vi "delete duplicates.vi"(9 "After Var Name":string[](array[string]), 10 "subscripts":string[](array[string]), 11 "Name":string[](array[string])) -> (0 "After Var Name Out":string[](array[string]), 1 "Full Names":string[][](array[string]), 2 "Subscripts Out":string[][](array[string]), 3 "Name Out":string[](array[string]), 4 "Name.Sub":string[](array[string]))   [LabVIEW 2015, in "AguaClara Library.lvlib"]
uses:
  ADT 2/AguaClara Library.lvlib
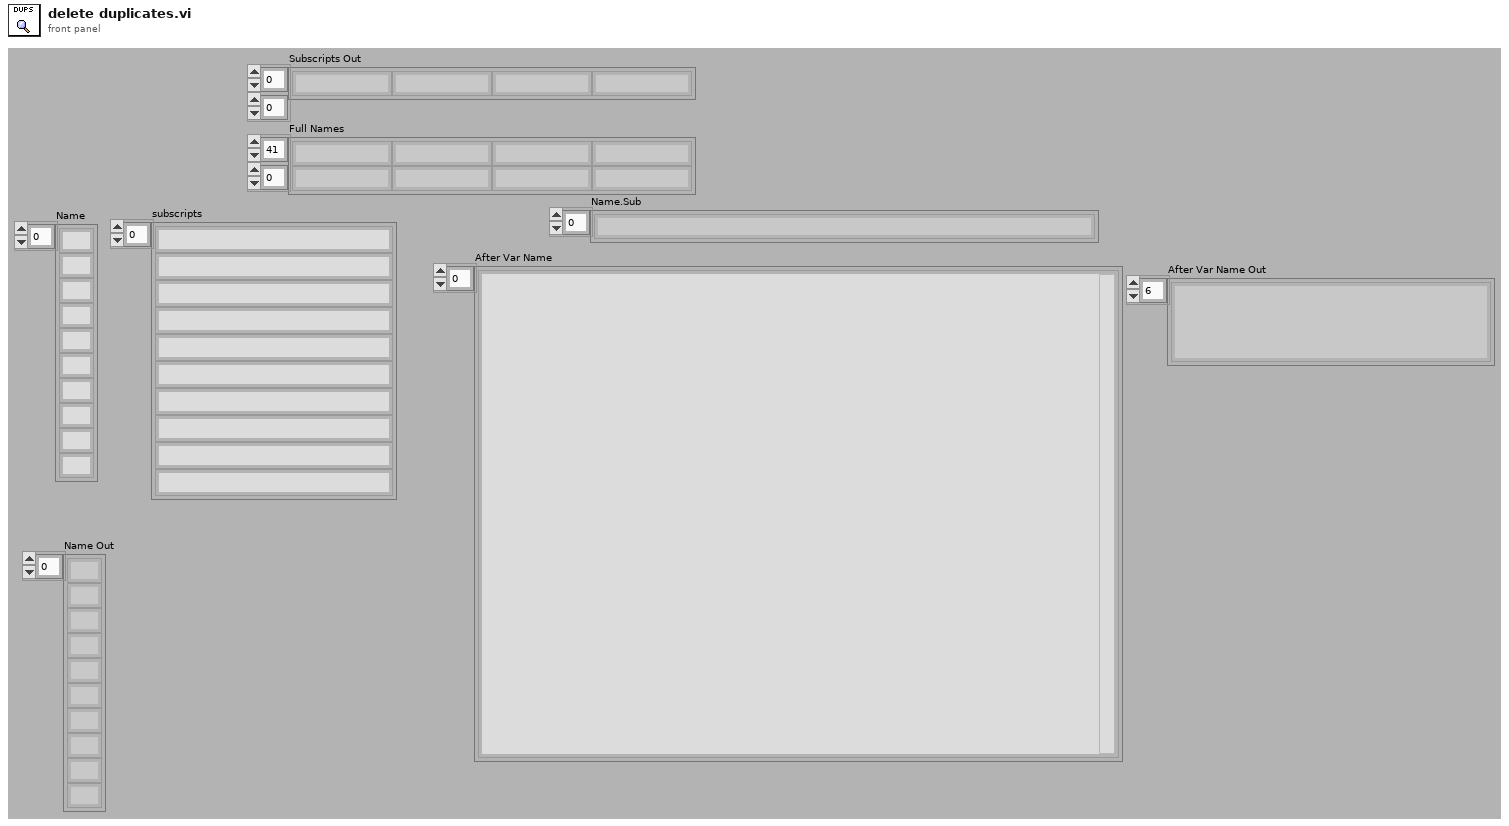
[diagram p1: front panel]
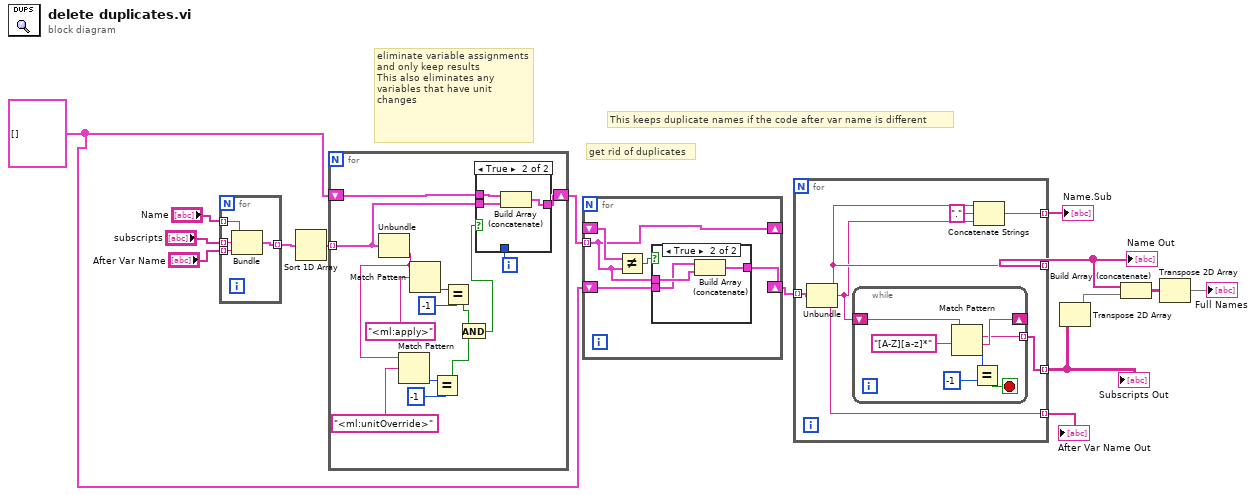
[diagram p0: block diagram]
diagram:
  w1 = cluster{string, string, "XML":string}[] []
  # "eliminate variable assignments and only keep results\nThis also eliminates any variables that have unit changes"
  # "This keeps duplicate names if the code after var name is different"
  # "get rid of duplicates"
  n1 = for {
    tunnel: "Name" -> [w19] mode=indexing
    tunnel: "subscripts" -> [w18] mode=indexing
    tunnel: [w17] -> w13 mode=indexing
    tunnel: "After Var Name" -> [w16] mode=indexing
    n2 = Bundle(w19, w18, "XML"=w16) -> (w17:cluster{string, string, "XML":string})  [unwired: 1 in]
  }
  n3 = Sort 1D Array(array=w13) -> (sorted array=w3:cluster{string, string, "XML":string}[])
  n4 = for {
    tunnel: w3 -> [w30] mode=indexing
    shift-right: [w29] -> w2
    shift-left: w1 -> [w28]
    i -> [w31]
    n5 = Unbundle(w30) -> ("XML"=w23:string)  [unwired: 2 out]
    n6 = Match Pattern(string=w23, regular expression="<ml:unitOverride>") -> (offset past match=w26:i32)  [unwired: 1 in, 3 out]
    n7 = Match Pattern(string=w23, regular expression="<ml:apply>") -> (offset past match=w33:i32)  [unwired: 1 in, 3 out]
    n8 = Equal?(x=w26, y=-1) -> (x = y?=w22:bool)
    n9 = Equal?(x=w33, y=-1) -> (x = y?=w21:bool)
    n10 = And(x=w21, y=w22) -> (x .and. y?=w20:bool)
    n11 = case shown="True" w20 {
      tunnel: w31 -> [_ _]
      tunnel: w30 -> [_ w37]
      tunnel: [w34 w36] -> w29
      tunnel: w28 -> [w34 w35]
      frame False {
      }
      frame True {
        n12 = Build Array (concatenate)(w35, w37) -> (w36:cluster{string, string, "XML":string}[])
      }
    }
  }
  n13 = for {
    tunnel: w2 -> [w41] mode=indexing
    shift-right: [w41] -> _
    shift-left: _ -> [w42]
    shift-right: [w40] -> w5
    shift-left: w1 -> [w39]
    n14 = Not Equal?(x=w42, y=w41) -> (x != y?=w38:bool)
    n15 = case shown="True" w38 {
      tunnel: w41 -> [_ w46]
      tunnel: [w43 w45] -> w40
      tunnel: w39 -> [w43 w44]
      frame False {
      }
      frame True {
        n16 = Build Array (concatenate)(w44, w46) -> (w45:cluster{string, string, "XML":string}[])
      }
    }
  }
  n17 = for {
    tunnel: w5 -> [w53] mode=indexing
    tunnel: [w50] -> w11 mode=indexing
    tunnel: [w52] -> w12 mode=indexing
    tunnel: [w51] -> w6 mode=indexing
    tunnel: [w47] -> w4 mode=indexing
    n18 = Unbundle(w53) -> (w50:string, w48:string, "XML"=w51:string)
    n19 = while {
      shift-right: [w55] -> _
      shift-left: w48 -> [w56]
      tunnel: [w54] -> w52 mode=indexing
      stop <- w58 stop-if-true
      n20 = Match Pattern(string=w56, regular expression="[A-Z][a-z]*" ("search string/char (-)")) -> (match substring=w54:string, after substring=w55:string, offset past match=w59:i32)  [unwired: 1 in, 1 out]
      n21 = Equal?(x=w59, y=-1) -> (x = y?=w58:bool)
    }
    n22 = Concatenate Strings(w50, "." ("string"), w48) -> (w47:string)
  }
  "Name Out" <- w11
  "Subscripts Out" <- w12
  "After Var Name Out" <- w6
  "Name.Sub" <- w4
  n23 = Transpose 2D Array(2D array=w12) -> (transposed array=w8:string[][])
  n24 = Build Array (concatenate)(w11, w8) -> (w10:string[][])
  n25 = Transpose 2D Array(2D array=w10) -> (transposed array=→"Full Names":string[][])
